vi "Main.vi"() -> ()   [LabVIEW 2014]
uses:
  <vilib>/myRIO/Instrument Drivers/Onboard IO/I2C/typedefs/I2C User Configuration.ctl
  <vilib>/myRIO/Instrument Drivers/Onboard IO/I2C/typedefs/I2C Transfer Rate.ctl
  <vilib>/myRIO/Common/Instrument Driver Framework/myRIO v1.0/UART/vis/myRIO v1.0 Close UART.vi
  <vilib>/Utility/error.llb/Error Cluster From Error Code.vi
  <vilib>/myRIO/Common/Instrument Driver Framework/Utilities/vis/FPGA Ref Manager.vi
  <vilib>/myRIO/Common/Instrument Driver Framework/myRIO v1.0/myRIO v1.0 Reset FPGA.vi
  <vilib>/myRIO/Common/Instrument Driver Framework/myRIO v1.0/IRQ/vis/myRIO v1.0 IRQ Info FGV.vi
  <vilib>/myRIO/Common/Instrument Driver Framework/myRIO v1.0/IRQ/vis/myRIO v1.0 Timer IRQ Info FGV.vi
  <vilib>/myRIO/Common/Instrument Driver Framework/myRIO v1.0/IRQ/vis/myRIO v1.0 ISR Agent.vi
  <vilib>/myRIO/Instrument Drivers/Utilities/Utilities.lvlib
  <vilib>/myRIO/Instrument Drivers/Onboard IO/I2C/I2C.lvlib
panel:
  out "Waveform Chart":i16(graph)
  out "x-rate":dbl
  out "Bytes Read 2":u8[](array[numeric])
  out "Bytes Read":u8[](array[numeric])
  out "error out":errorcluster
  in  "Stop Button":bool
  # "Overview: The myRIO Project template acquires acceleration data from the onboard accelerometer and displays the changes of acceleration values in a waveform chart.\nInstructions:\n1. Check the myRIO target IP Address in the project and make sure the target IP Address is correct. \n2. Run the VI."
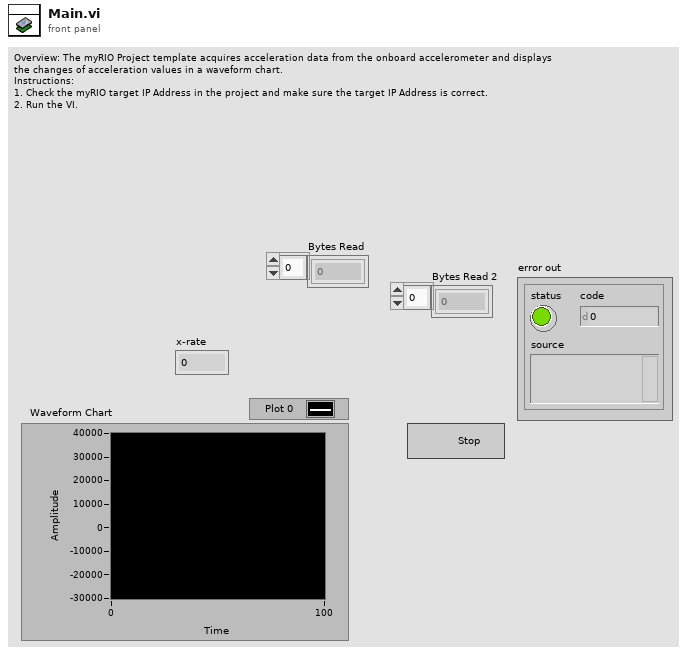
[diagram p1: front panel]
types:
  T1 = typedef "I2C.lvlib/I2C User Configuration.ctl" = cluster{"I2C Transfer Rate":T2}
  T2 = typedef "I2C.lvlib/I2C Transfer Rate.ctl" = enum16{"Standard mode (100 kbps)", "Fast mode (400 kbps)"}
  T3 = typedef "I2C.lvlib/I2C Reference.ctl" = cluster{"myRIO Reference":T4, "I2C Channels Enum":T8, "I2C Configuration":T9}
  T4 = typedef "myRIO Generic Hardware Reference.ctl" = cluster{"myRIO Model":T5, "myRIO Hardware Reference":T6}
  T5 = typedef "Hardware Version Enum.ctl" = enum16{"Unknown", "myRIO-1900", "myRIO-1950"}
  T6 = typedef "myRIO v1.0 Reference.ctl" = cluster{"Generic FPGA Reference":T7, "Allow multiple opens":bool}
  T7 = typedef "Generic FPGA Reference.ctl" = refnum<k20>
  T8 = typedef "I2C Channels Enum.ctl" = enum16{"Not Connected", "A/I2C", "B/I2C"}
  T9 = typedef "I2C.lvlib/I2C Configuration.ctl" = cluster{"I2C Transfer Rate":T2}
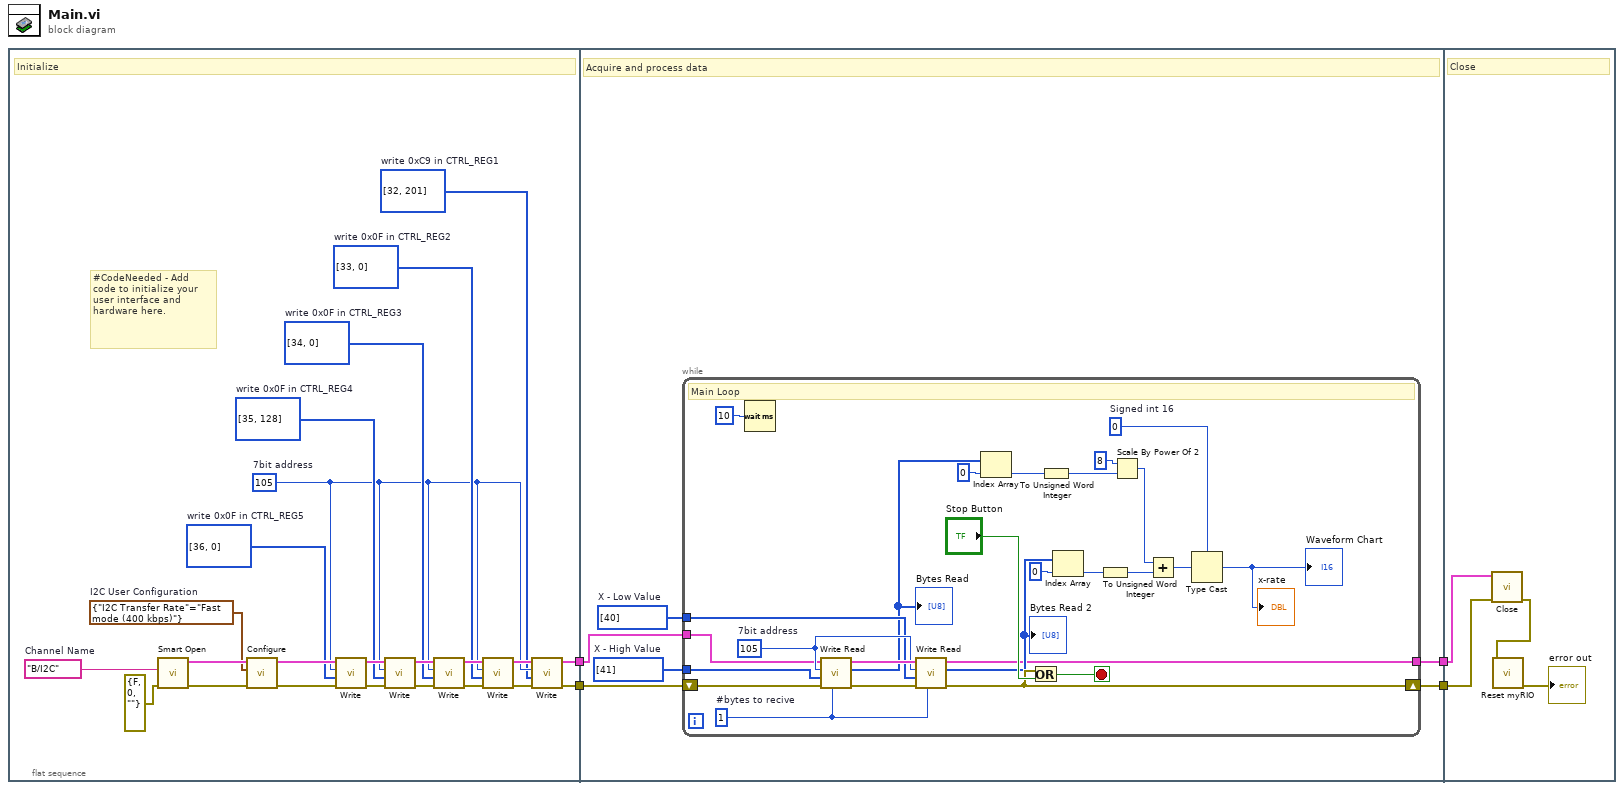
[diagram p0: block diagram]
diagram:
  n1 = flat-sequence {
    tunnel: [w6] -> w3
    tunnel: [w5] -> w2
    tunnel: [w33] -> w4
    tunnel: w3 -> [w30]
    tunnel: w2 -> [w29]
    tunnel: [w28] -> w1
    tunnel: w4 -> [w61]
    tunnel: w1 -> [w62]
    frame #0 {
      w9 = u8 105  # 7bit address
      w20 = u8[] [36, 0]  # write 0x0F in CTRL_REG5
      w18 = u8[] [35, 128]  # write 0x0F in CTRL_REG4
      w15 = u8[] [34, 0]  # write 0x0F in CTRL_REG3
      w12 = u8[] [33, 0]  # write 0x0F in CTRL_REG2
      w8 = u8[] [32, 201]  # write 0xC9 in CTRL_REG1
      w23 = T1 {"I2C Transfer Rate"=enum."Fast mode (400 kbps)"}  # I2C User Configuration
      w27 = tag "B/I2C"  # Channel Name
      # "#CodeNeeded - Add code to initialize your user interface and hardware here."
      # "Initialize"
      n2 = call <vilib>:"Smart Open.vi"("error in (no error)"=errorcluster {"status"=FALSE, "code"=0, "source"=""} ("error out"), "Channel Name"=w27) -> ("error out"=w25:errorcluster, "I2C Ref Out"=w24:T3)  [unwired: 8 in]
      n3 = call <vilib>:"Configure.vi"("error in (no error)"=w25, "I2C User Configuration"=w23, "I2C Ref In"=w24) -> ("error out"=w21:errorcluster, "I2C Ref Out"=w22:T3)  [unwired: 7 in]
      n4 = call <vilib>:"Write.vi"("error in (no error)"=w21, "Bytes to Write"=w20, "Slave Address (7-bit)"=w9, "I2C Ref In"=w22) -> ("error out"=w17:errorcluster, "I2C Ref Out"=w19:T3)  [unwired: 6 in]
      n5 = call <vilib>:"Write.vi"("error in (no error)"=w17, "Bytes to Write"=w18, "Slave Address (7-bit)"=w9, "I2C Ref In"=w19) -> ("error out"=w14:errorcluster, "I2C Ref Out"=w16:T3)  [unwired: 6 in]
      n6 = call <vilib>:"Write.vi"("error in (no error)"=w14, "Bytes to Write"=w15, "Slave Address (7-bit)"=w9, "I2C Ref In"=w16) -> ("error out"=w11:errorcluster, "I2C Ref Out"=w13:T3)  [unwired: 6 in]
      n7 = call <vilib>:"Write.vi"("error in (no error)"=w11, "Bytes to Write"=w12, "Slave Address (7-bit)"=w9, "I2C Ref In"=w13) -> ("error out"=w7:errorcluster, "I2C Ref Out"=w10:T3)  [unwired: 6 in]
      n8 = call <vilib>:"Write.vi"("error in (no error)"=w7, "Bytes to Write"=w8, "Slave Address (7-bit)"=w9, "I2C Ref In"=w10) -> ("error out"=w6:errorcluster, "I2C Ref Out"=w5:T3)  [unwired: 6 in]
    }
    frame #1 {
      w31 = u8[] [40]  # X - Low Value
      w32 = u8[] [41]  # X - High Value
      # "Acquire and process data"
      n9 = while {
        shift-right: [w53] -> w33
        shift-left: w30 -> [w56]
        tunnel: w32 -> [w55]
        tunnel: w31 -> [w49]
        tunnel: w29 -> [w48]
        tunnel: [w34] -> w28
        stop <- w58 stop-if-true
        w46 = i16 0  # Signed int 16
        w51 = u8 1  # #bytes to recive
        w50 = u8 105  # 7bit address
        # "Main Loop"
        n10 = Wait (ms)(milliseconds to wait=u32 10) -> ()  [unwired: 1 out]
        n11 = call <vilib>:"Write Read.vi"("Byte Count"=w51, "error in (no error)"=w56, "Bytes to Write"=w55, "Slave Address (7-bit)"=w50, "I2C Ref In"=w48) -> ("error out"=w54:errorcluster, "Bytes Read"=w36:u8[], "I2C Ref Out"=w52:T3)  [unwired: 3 in]
        "Bytes Read" <- w36
        n12 = call <vilib>:"Write Read.vi"("Byte Count"=w51, "error in (no error)"=w54, "Bytes to Write"=w49, "Slave Address (7-bit)"=w50, "I2C Ref In"=w52) -> ("error out"=w53:errorcluster, "Bytes Read"=w37:u8[], "I2C Ref Out"=w34:T3)  [unwired: 3 in]
        "Bytes Read 2" <- w37
        n13 = Index Array(array=w36, index=0) -> (element=w45:u8)
        n14 = Or(x=w53, y="Stop Button") -> (x .or. y?=w58:bool)
        n15 = To Unsigned Word Integer(number=w45) -> (unsigned 16bit integer=w43:u16)
        n16 = Index Array(array=w37, index=0) -> (element=w40:u8)
        n17 = To Unsigned Word Integer(number=w40) -> (unsigned 16bit integer=w39:u16)
        n18 = Scale By Power Of 2(n=i16 8, x=w43) -> (x*2^n=w41:u16)
        n19 = Add(x=w41, y=w39) -> (x+y=w38:u16)
        n20 = Type Cast(type=w46, x=w38) -> (*(type *) &x=→"x-rate" →"Waveform Chart":i16)
      }
    }
    frame #2 {
      # "Close"
      n21 = call <vilib>:"Close.vi"("error in (no error)"=w61, "I2C Ref In"=w62) -> ("error out"=w60:errorcluster)  [unwired: 9 in]
      n22 = call <vilib>:"Reset myRIO.vi"("error in (no error)"=w60) -> ("error out"=→"error out":errorcluster)  [unwired: 10 in]
    }
  }
